vi "MAIN_cRIO_ZNB_AMI.vi"() -> ()   [LabVIEW 2017]
doc: "Use this template to build a producer/consumer design pattern with events to produce queue items. Use this design pattern instead of the user interface event handler pattern for user interfaces when you want to execute code asynchronously in response to an event without slowing the user interface responsiveness."
uses:
  MEDIDA_cRIO_ZNB_AMI_DATOS.ctl
  AMI MAGNET/Status AMI.ctl
  MAIN_cRIO_ZNB_AMI.ctl
  DISPLAY/UserEventData.ctl
  DISPLAY/DataType.ctl
  cRIO_ZNB_AMI_GLOBALES.vi
panel:
  out "X state":T1=1 items=["Unknown", "RAMPING to target field/current", "HOLDING at the target field/current", "PAUSED", "Ramping in MANUAL UP mode", "Ramping in MANUAL DOWN mode", "ZEROING CURRENT (in progress)", "Quench detected", "At ZERO current", "Heating persistent switch", "Cooling persistent switch", "External Rampdown active"]
  out "Y state":T1=1 items=["Unknown", "RAMPING to target field/current", "HOLDING at the target field/current", "PAUSED", "Ramping in MANUAL UP mode", "Ramping in MANUAL DOWN mode", "ZEROING CURRENT (in progress)", "Quench detected", "At ZERO current", "Heating persistent switch", "Cooling persistent switch", "External Rampdown active"]
  out "Z state":T1=1 items=["Unknown", "RAMPING to target field/current", "HOLDING at the target field/current", "PAUSED", "Ramping in MANUAL UP mode", "Ramping in MANUAL DOWN mode", "ZEROING CURRENT (in progress)", "Quench detected", "At ZERO current", "Heating persistent switch", "Cooling persistent switch", "External Rampdown active"]
  out "Temperature Status":i32(ring) items=["TemperatureUnknown", "Stable", "Tracking", "Near"]
  out "DataPath":path
  out "XY Graph 4":cluster{dbl[], dbl[]}[](graph)
  out "XY Graph 3":cluster{dbl[], dbl[]}[](graph)
  out "XY Graph 2":cluster{dbl[], dbl[]}[](graph)
  out "XY Graph 1":cluster{dbl[], dbl[]}[](graph)
  out "arrayDatos":T2[](array[typedef]) {"CampoZ(T)" format="%.3e"; "CampoY(T)" format="%.3e"; "A.Input3(V)" format="%.3e"; "A.Input4(V)" format="%.3e"; "A.Input1(V)" format="%.3e"; "A.Input2(V)" format="%.3e"; "Temperatura(K)" format="%.3e"; "CampoX(T)" format="%.3e"; "Tiempo(min)" format="%.3e"}
  out "Puntos":i32=10000
  out "Status":bool
  in  "Programa":i32(listbox)=-1
  in  "Setup":bool
  in  "Programar":bool
  in  "Fin":bool
  in  "Auto":bool
  in  "Parar":bool
  out "Tiempo(min)":dbl format="%.2f"
  out "A.Input2(V)":dbl format="%.3f"
  out "A.Input3(V)":dbl format="%.3f"
  out "A.Input4(V)":dbl format="%.3f"
  out "Campo Mag(T)":dbl format="%.2f"
  out "Temperatura(K)":dbl format="%.2f"
  out "TotalSeq":string[](array[string])
  in  "Grafica":T3(ring)
  out "Estado":string
  out "NumCommando":string
  in  "Pausa":bool
  in  "Saltar":bool
  out "Total Comandos":i32
  out "Comando actual":i32
  out "Datos":T2 {"CampoZ(T)" format="%.3e"; "CampoY(T)" format="%.3e"; "A.Input3(V)" format="%.3e"; "A.Input4(V)" format="%.3e"; "A.Input1(V)" format="%.3e"; "A.Input2(V)" format="%.3e"; "Temperatura(K)" format="%.3e"; "CampoX(T)" format="%.3e"; "Tiempo(min)" format="%.3e"}
  out "error out":errorcluster
  # "cRIO - 9074.ZNB.AMI\nEnero 2023 V1.0  a-sslcdms LV2017"
  # "Secuencia en marcha. Pulsar para PAUSAR"
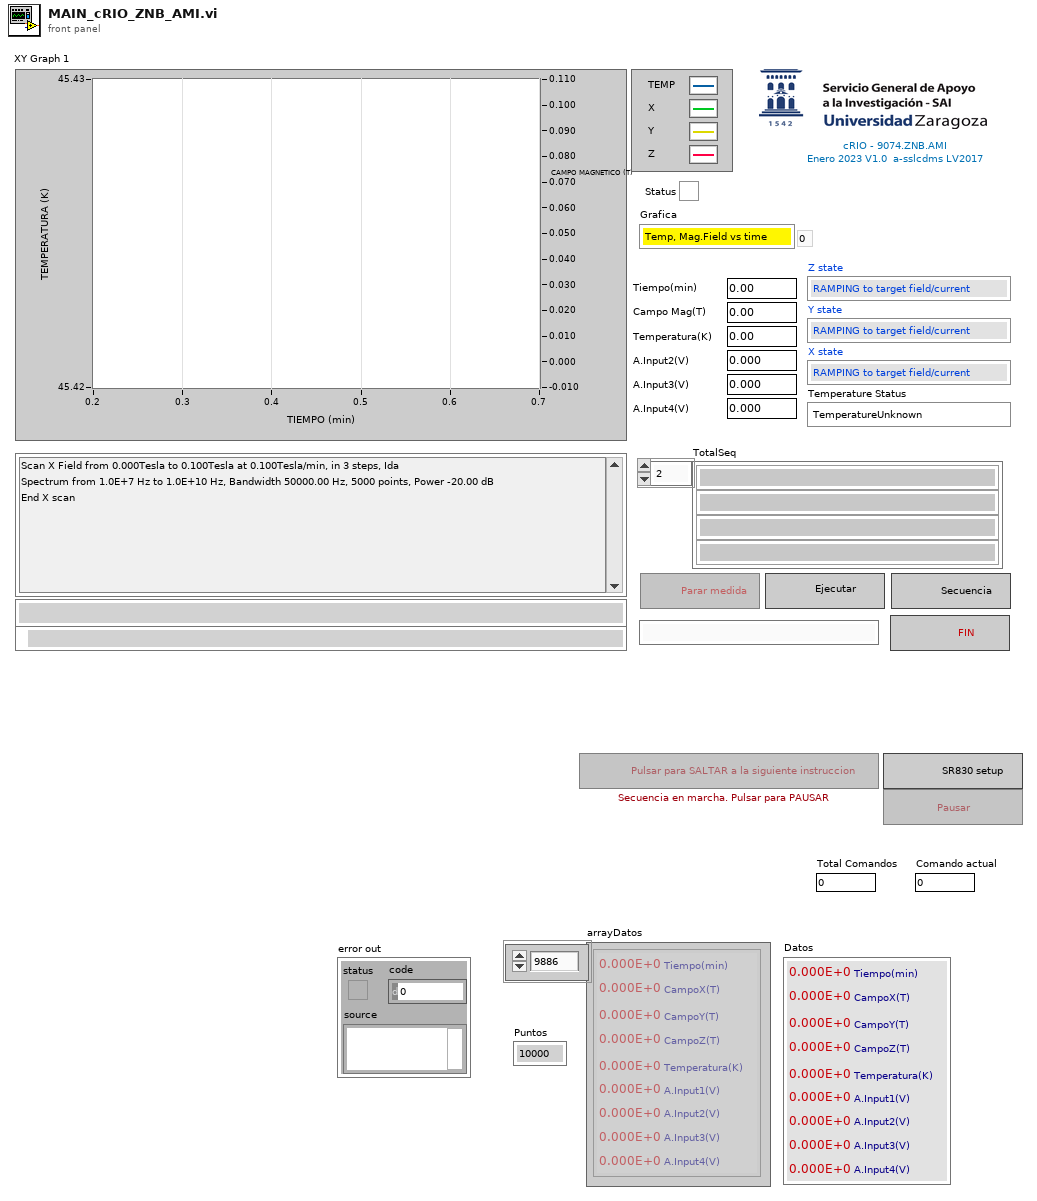
[diagram p1: front panel]
types:
  T1 = typedef "Status AMI.ctl" = u16
  T2 = typedef "MEDIDA_cRIO_ZNB_AMI_DATOS.ctl" = cluster{"Tiempo(min)":dbl, "CampoX(T)":dbl, "CampoY(T)":dbl, "CampoZ(T)":dbl, "Temperatura(K)":dbl, "A.Input1(V)":dbl, "A.Input2(V)":dbl, "A.Input3(V)":dbl, "A.Input4(V)":dbl}
  T3 = enum16{"Temp, Mag.Field vs time", "Voltajes 2,3,4 vs Tiempo", "Voltajes 2,3,4 vs Campo", "Voltajes 2,3,4 vs Temper."}
  T4 = typedef "UserEventData.ctl" = cluster{"DataType":T5, "Data":variant}
  T5 = typedef "DataType.ctl" = enum16{"Initialize Front Panel", "Update Front Panel", "Update Graph", "Enable/Disable Controls", "Update Status"}
  T6 = typedef "MAIN_cRIO_ZNB_AMI.ctl" = enum16{"Inicializar", "Ajustes", "Medir", "Finalizar"}
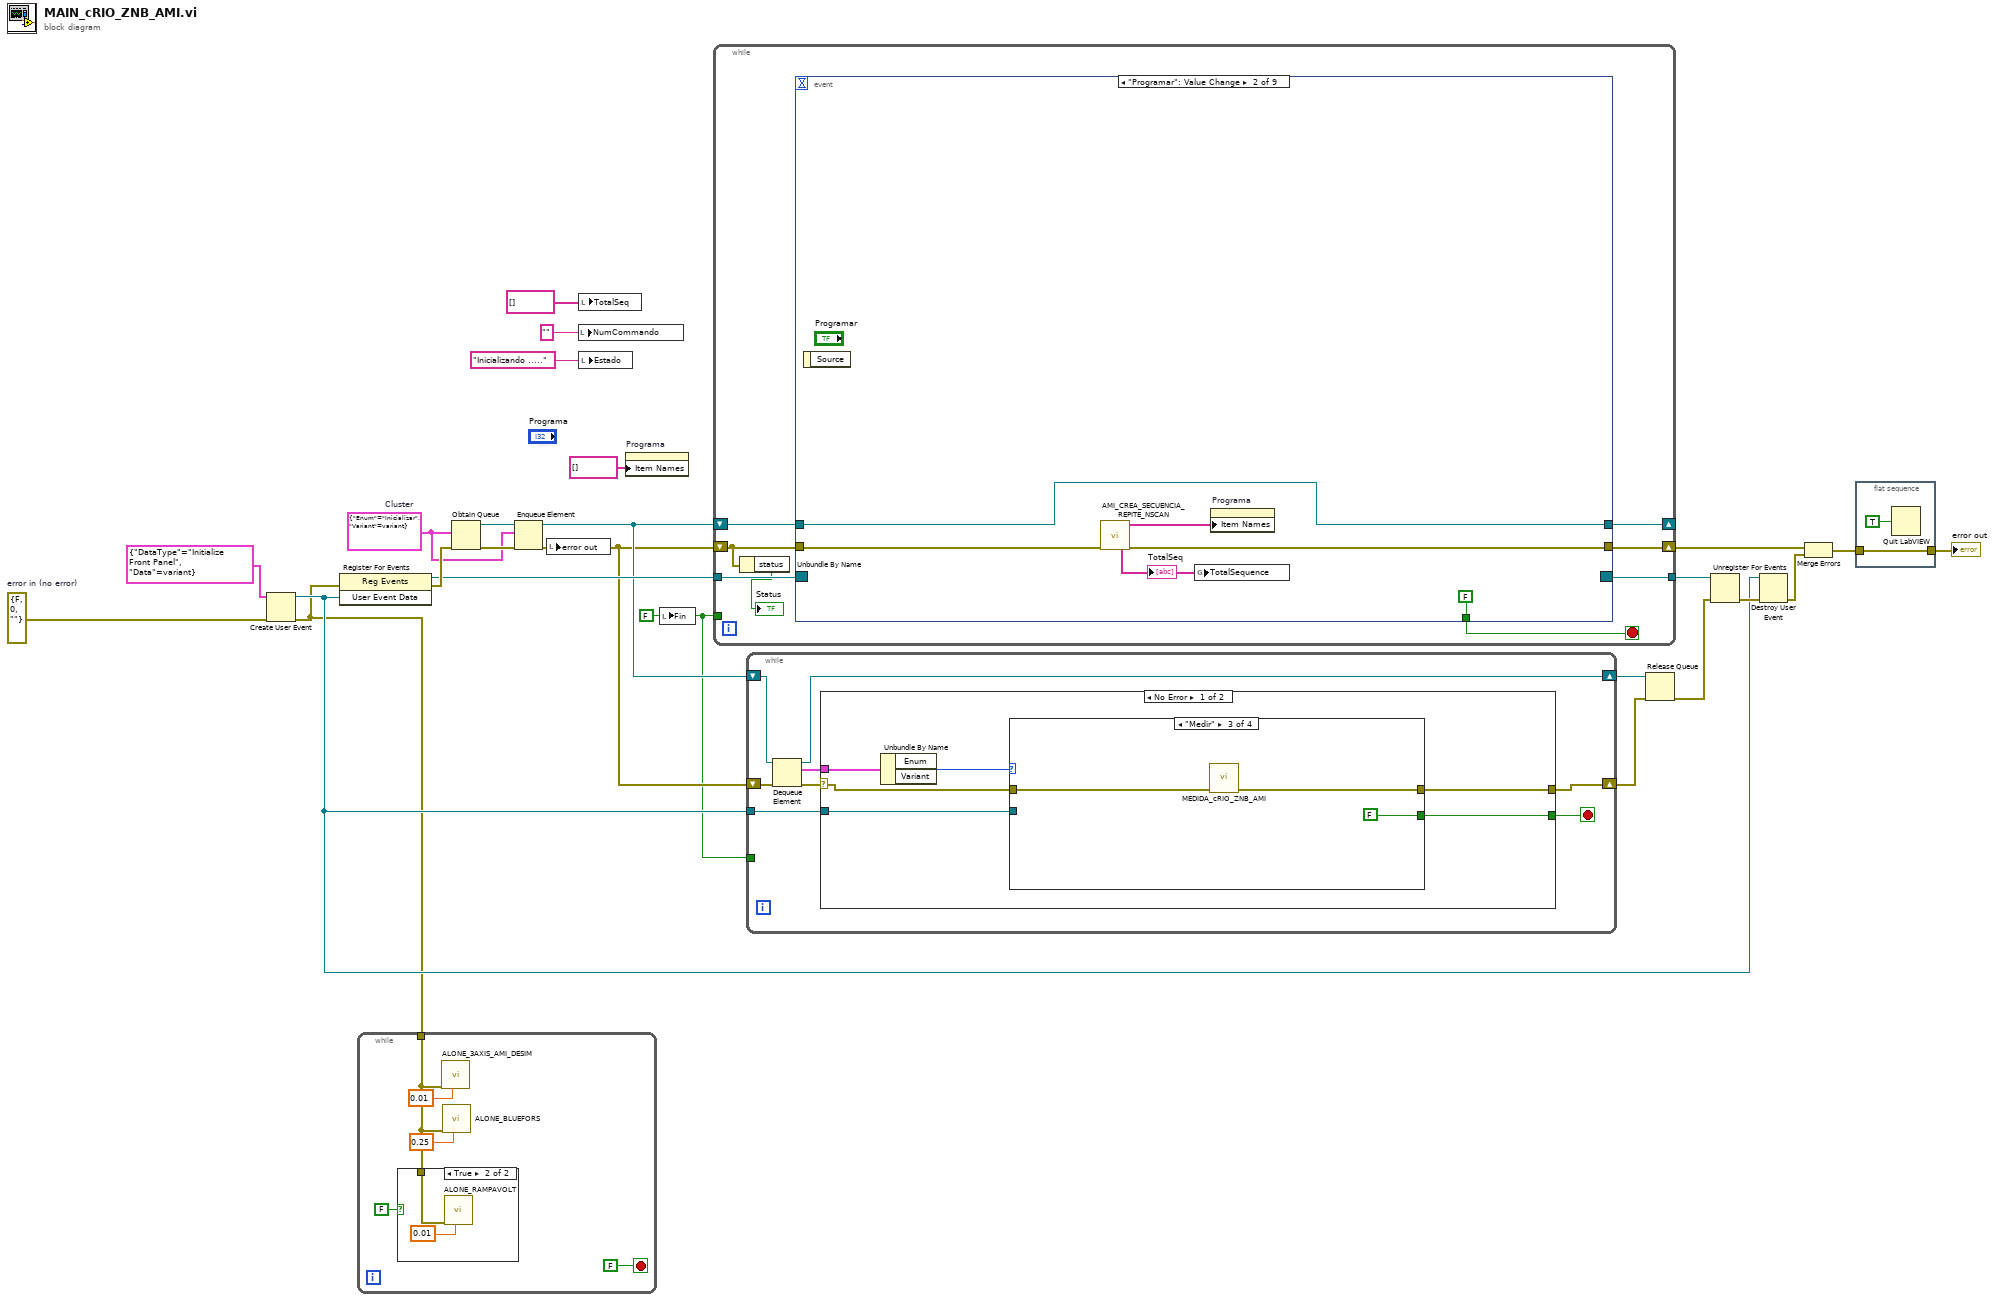
[diagram p0: block diagram]
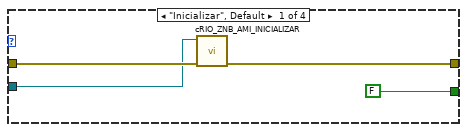
[diagram p3: hidden frame]
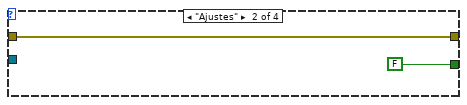
[diagram p4: hidden frame]
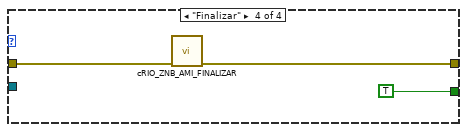
[diagram p5: hidden frame]
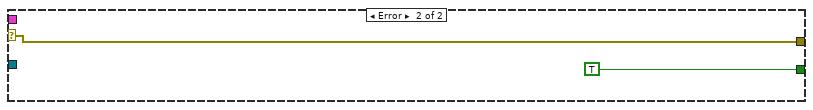
[diagram p6: hidden frame]
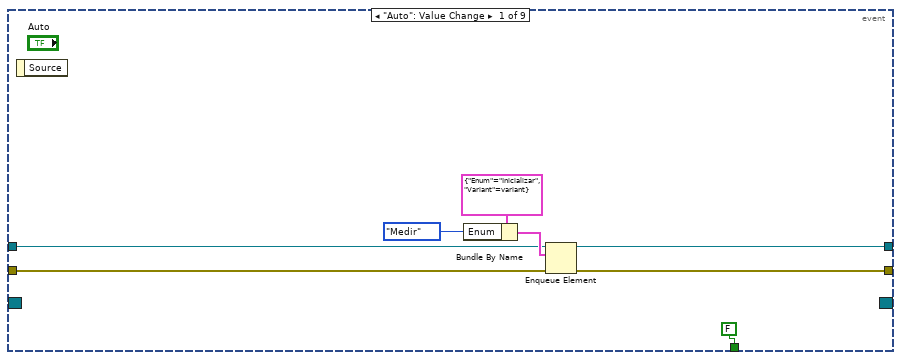
[diagram p7: hidden frame]
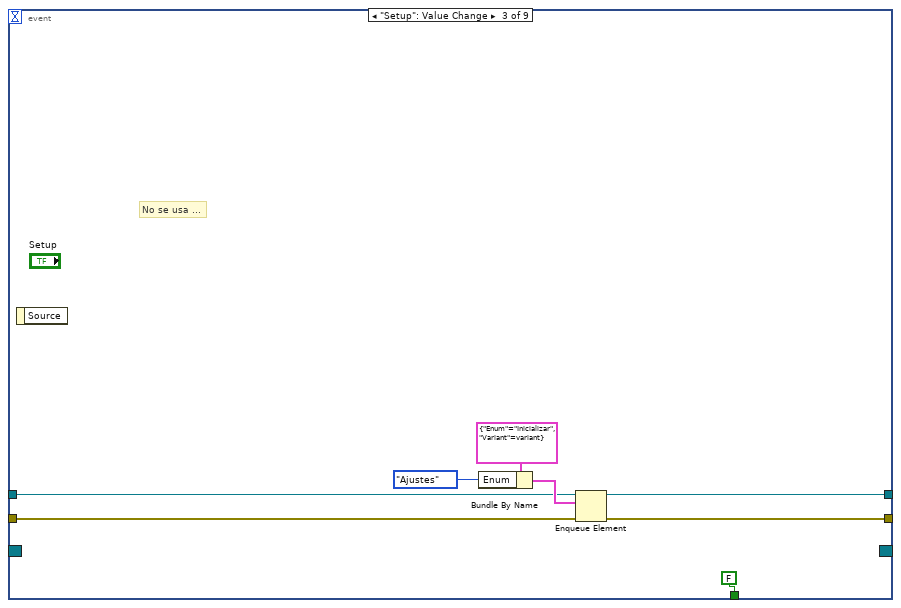
[diagram p8: hidden frame]
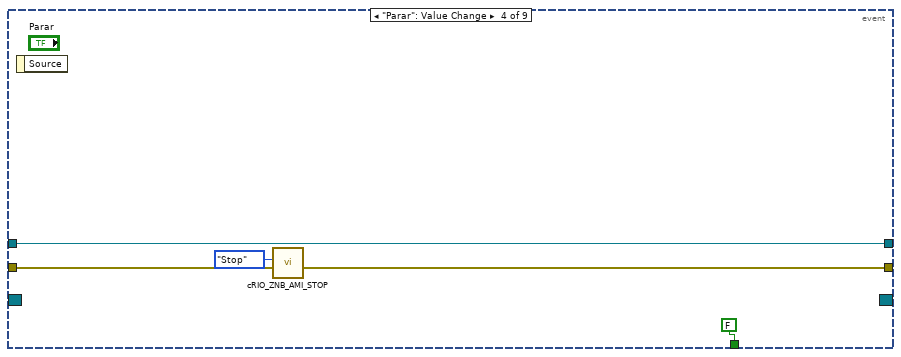
[diagram p9: hidden frame]
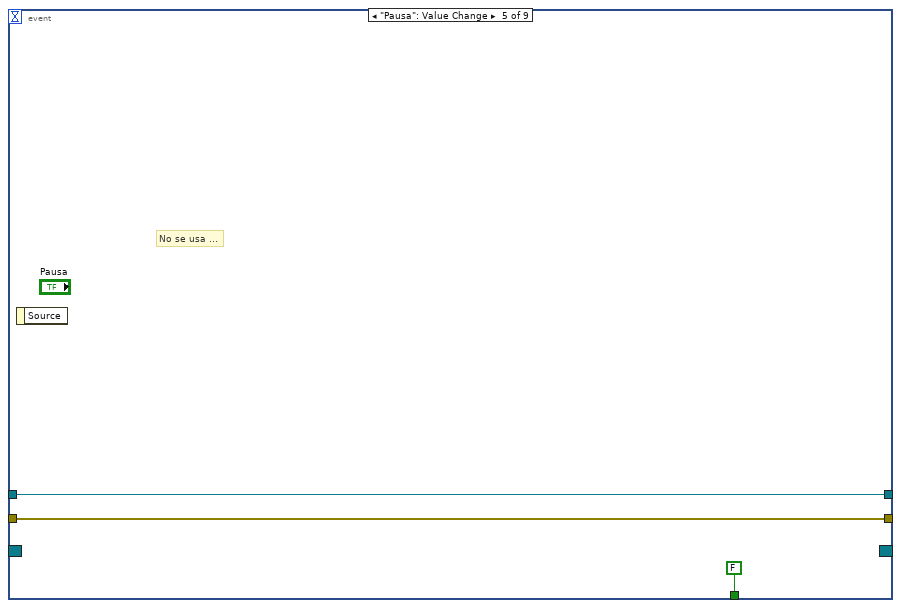
[diagram p10: hidden frame]
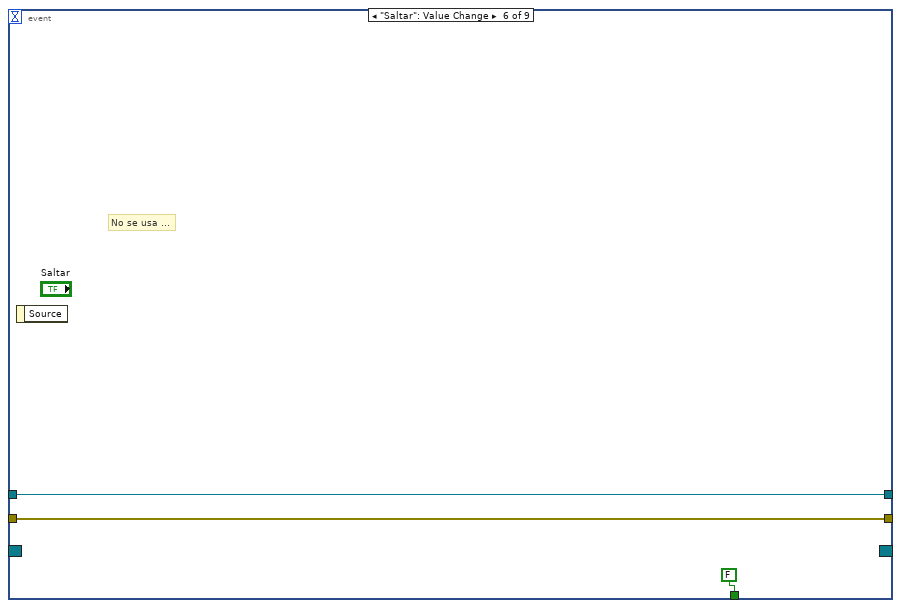
[diagram p11: hidden frame]
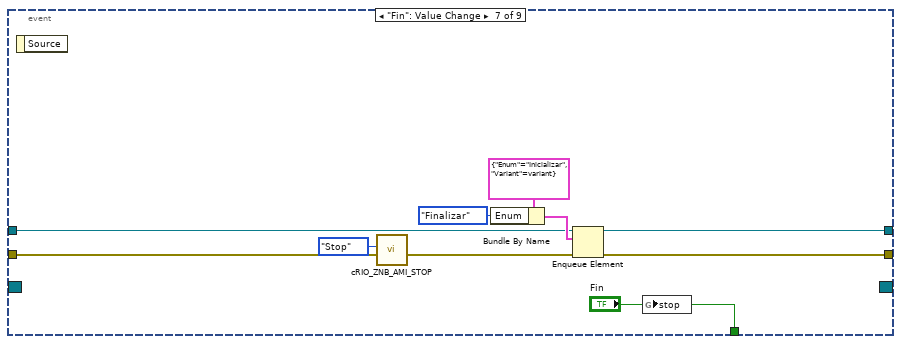
[diagram p12: hidden frame]
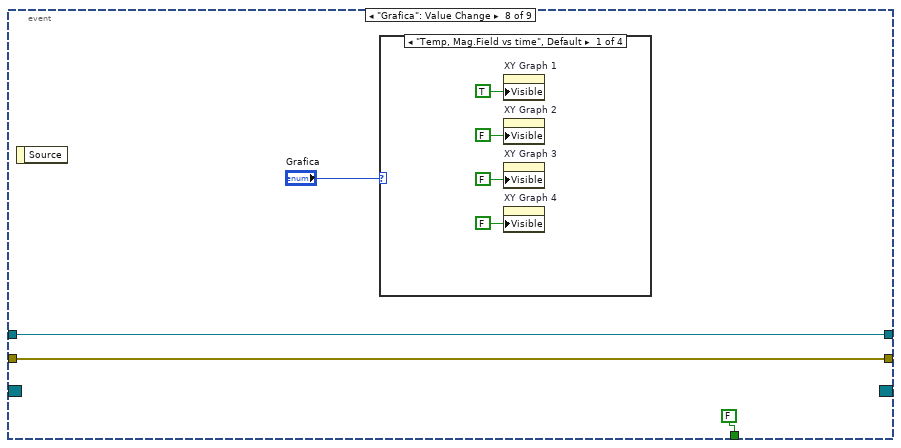
[diagram p13: hidden frame]
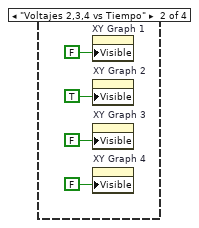
[diagram p14: hidden frame]
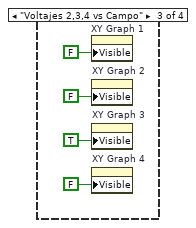
[diagram p15: hidden frame]
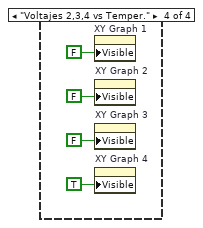
[diagram p16: hidden frame]
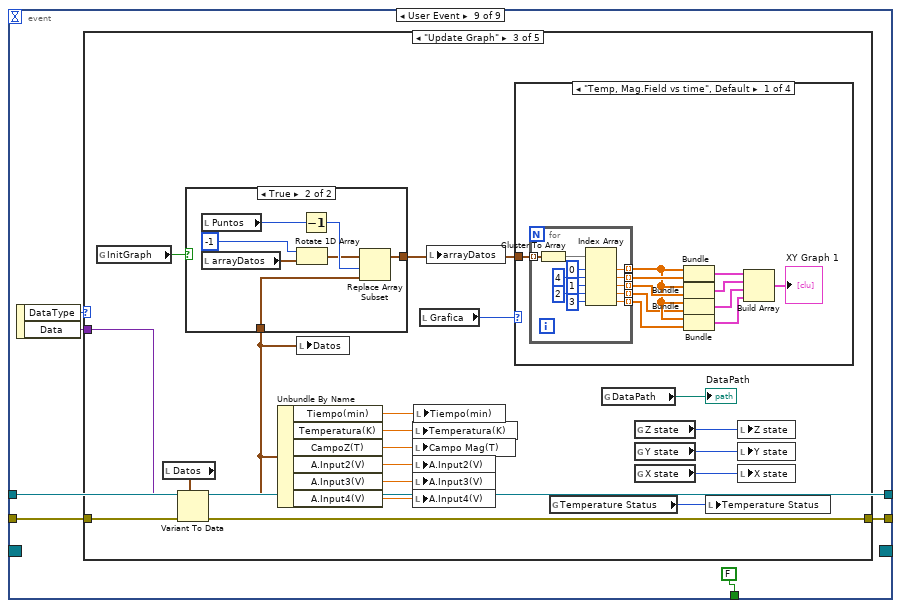
[diagram p17: hidden frame]
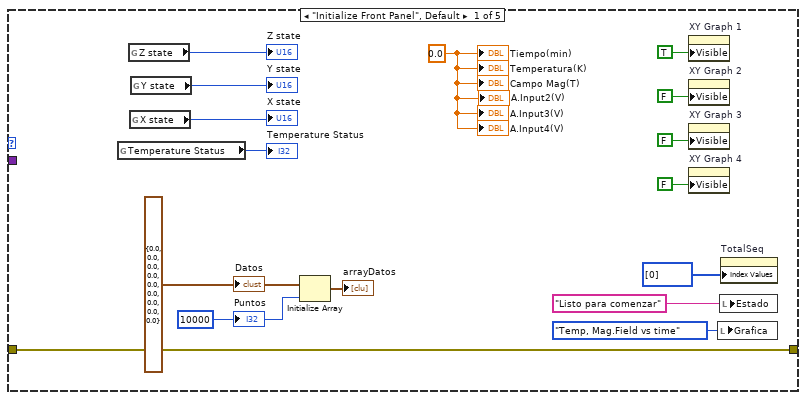
[diagram p18: hidden frame]
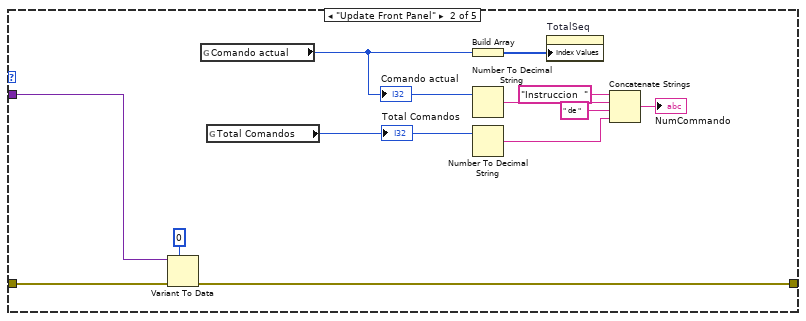
[diagram p19: hidden frame]
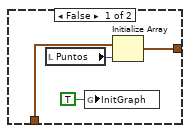
[diagram p20: hidden frame]
diagram:
  w5 = FALSE ("Fin")
  w2 = errorcluster {"status"=FALSE, "code"=0, "source"=""}  # error in (no error)
  w23 = cluster{"Enum":T6, "Variant":variant} {"Enum"=enum."Inicializar", "Variant"=variant}  # Cluster
  n1 = Create User Event(user event datatype=T4 {"DataType"=enum."Initialize Front Panel", "Data"=variant} ("User Event Data"), error in=w2) -> (user event=w11:refnum<user-event>, error out=w1:errorcluster)
  n2 = register-events(error in=w1, w11) -> (reference out=w15:refnum<event-registration>, error out=w25:errorcluster)  [unwired: 1 in]
  n3 = while {
    tunnel: w1 -> [w30]
    stop <- FALSE stop-if-true
    n4 = case shown="True" FALSE {
      tunnel: w30 -> [_ w32]
      frame False {
      }
      frame True {
        n5 = call "ALONE_RAMPAVOLT.vi"("Refresco(s)"=0.01, "error in (no error)"=w32) -> ()  [unwired: 8 in, 2 out]
      }
    }
    n6 = call "ALONE_3AXIS_AMI_DESIM.vi"("Refresco(s)"=0.01, "error in (no error)"=w30) -> ()  [unwired: 8 in, 2 out]
    n7 = call "ALONE_BLUEFORS.vi"("Refresco(s)"=0.25, "error in (no error)"=w30) -> ()  [unwired: 9 in, 1 out]
  }
  n8 = Obtain Queue(element data type=w23, error in (no error)=w25) -> (queue out=w22:refnum<queue>, error out=w24:errorcluster)  [unwired: 3 in, 1 out]
  n9 = Enqueue Element(queue=w22, element=w23, error in (no error)=w24) -> (queue out=w13:refnum<queue>, error out=w12:errorcluster)  [unwired: 1 in, 1 out]
  n10 = local write "error out"(w12) -> ()
  n11 = local write "NumCommando"("" ("NumCommando")) -> ()
  n12 = local write "TotalSeq"(string[] [] ("TotalSequence")) -> ()
  n13 = local write "Estado"("Inicializando ....." ("String")) -> ()
  n14 = property on="Programa" class="LstBox (strict)"("Item Names"=string[] []) -> ()  [unwired: 2 in, 2 out]
  n15 = local write "Fin"(w5) -> ()
  n16 = while {
    shift-right: [w35] -> w18
    shift-left: w12 -> [w34]
    shift-right: [w39] -> _
    shift-left: w13 -> [w40]
    tunnel: w15 -> [w37]
    tunnel: [w36] -> w14
    tunnel: w5 -> [_]
    stop <- w38 stop-if-true
    n17 = Unbundle By Name(w34) -> ("status"=→"Status":bool)
    n18 = event shown="[1] \"Programar\": Value Change" {
      selector: w37 -> [_ _ _ _ _ _ _ _ _]
      dyn-events: [_ _ _ _ _ _ _ _ _] -> w36
      timeout: _ -> [_ _ _ _ _ _ _ _ _]
      tunnel: w40 -> [w43 w51 w55 w64 w69 w72 w78 w85 w105]
      tunnel: [w44 w51 w57 w64 w69 w72 w79 w85 w105] -> w39
      tunnel: w34 -> [w42 w53 w56 w66 w68 w71 w76 w84 w107]
      tunnel: [w45 w52 w58 w63 w68 w71 w80 w84 w106] -> w35
      tunnel: [FALSE ("Parar") FALSE ("Parar") FALSE ("Parar") FALSE ("Parar") FALSE ("Parar") FALSE ("Parar") "Fin" FALSE ("Parar") FALSE ("Parar")] -> w38
      event "Auto": Value Change {
        n19 = event-data() -> ()  [unwired: 1 in, 1 out]
        n20 = Bundle By Name(cluster=cluster{"Enum":T6, "Variant":variant} {"Enum"=enum."Inicializar", "Variant"=variant} ("Cluster"), "Enum"=MAIN_cRIO_ZNB_AMI."Medir") -> (w46:cluster{"Enum":T6, "Variant":variant})
        n21 = Enqueue Element(queue=w43, element=w46, error in (no error)=w42) -> (queue out=w44:refnum<queue>, error out=w45:errorcluster)  [unwired: 1 in, 1 out]
      }
      event "Programar": Value Change {
        n22 = event-data() -> ()  [unwired: 1 in, 1 out]
        n23 = call "AMI_CREA_SECUENCIA_REPITE_NSCAN.vi"("error in (no error)"=w53) -> ("error out"=w52:errorcluster, "SECUENCIA"=w50:string[], "TOTAL_REPS"=w49:string[])  [unwired: 7 in, 1 out]
        "TotalSeq" <- w49
        n24 = global write "cRIO_ZNB_AMI_GLOBALES.vi" "TotalSequence"(w49) -> ()
        n25 = property on="Programa" class="LstBox (strict)"("Item Names"=w50) -> ()  [unwired: 2 in, 2 out]
      }
      event "Setup": Value Change {
        # "No se usa ..."
        n26 = event-data() -> ()  [unwired: 1 in, 1 out]
        n27 = Bundle By Name(cluster=cluster{"Enum":T6, "Variant":variant} {"Enum"=enum."Inicializar", "Variant"=variant} ("Cluster"), "Enum"=MAIN_cRIO_ZNB_AMI."Ajustes") -> (w59:cluster{"Enum":T6, "Variant":variant})
        n28 = Enqueue Element(queue=w55, element=w59, error in (no error)=w56) -> (queue out=w57:refnum<queue>, error out=w58:errorcluster)  [unwired: 1 in, 1 out]
      }
      event "Parar": Value Change {
        n29 = event-data() -> ()  [unwired: 1 in, 1 out]
        n30 = call "cRIO_ZNB_AMI_STOP.vi"("error in (no error)"=w66, "Stop"=enum16{"Continue", "Stop", "Default"}."Stop") -> ("error out"=w63:errorcluster)  [unwired: 8 in, 1 out]
      }
      event "Pausa": Value Change {
        # "No se usa ..."
        n31 = event-data() -> ()  [unwired: 1 in, 1 out]
      }
      event "Saltar": Value Change {
        # "No se usa ..."
        n32 = event-data() -> ()  [unwired: 1 in, 1 out]
      }
      event "Fin": Value Change {
        n33 = event-data() -> ()  [unwired: 1 in, 1 out]
        n34 = call "cRIO_ZNB_AMI_STOP.vi"("error in (no error)"=w76, "Stop"=enum16{"Continue", "Stop", "Default"}."Stop") -> ("error out"=w75:errorcluster)  [unwired: 8 in, 1 out]
        n35 = Bundle By Name(cluster=cluster{"Enum":T6, "Variant":variant} {"Enum"=enum."Inicializar", "Variant"=variant} ("Cluster"), "Enum"=MAIN_cRIO_ZNB_AMI."Finalizar") -> (w81:cluster{"Enum":T6, "Variant":variant})
        n36 = Enqueue Element(queue=w78, element=w81, error in (no error)=w75) -> (queue out=w79:refnum<queue>, error out=w80:errorcluster)  [unwired: 1 in, 1 out]
        n37 = global write "cRIO_ZNB_AMI_GLOBALES.vi" "stop"("Fin") -> ()
      }
      event "Grafica": Value Change {
        n38 = event-data() -> ()  [unwired: 1 in, 1 out]
        n39 = case shown="\"Temp, Mag.Field vs time\", Default" "Grafica" {
          frame "Temp, Mag.Field vs time", Default {
            n40 = property on="XY Graph 1" class="XYGraph (strict)"("Visible"=TRUE) -> ()  [unwired: 2 in, 2 out]
            n41 = property on="XY Graph 2" class="XYGraph (strict)"("Visible"=FALSE) -> ()  [unwired: 2 in, 2 out]
            n42 = property on="XY Graph 3" class="XYGraph (strict)"("Visible"=FALSE) -> ()  [unwired: 2 in, 2 out]
            n43 = property on="XY Graph 4" class="XYGraph (strict)"("Visible"=FALSE) -> ()  [unwired: 2 in, 2 out]
          }
          frame "Voltajes 2,3,4 vs Tiempo" {
            n44 = property on="XY Graph 1" class="XYGraph (strict)"("Visible"=FALSE) -> ()  [unwired: 2 in, 2 out]
            n45 = property on="XY Graph 2" class="XYGraph (strict)"("Visible"=TRUE) -> ()  [unwired: 2 in, 2 out]
            n46 = property on="XY Graph 3" class="XYGraph (strict)"("Visible"=FALSE) -> ()  [unwired: 2 in, 2 out]
            n47 = property on="XY Graph 4" class="XYGraph (strict)"("Visible"=FALSE) -> ()  [unwired: 2 in, 2 out]
          }
          frame "Voltajes 2,3,4 vs Campo" {
            n48 = property on="XY Graph 1" class="XYGraph (strict)"("Visible"=FALSE) -> ()  [unwired: 2 in, 2 out]
            n49 = property on="XY Graph 2" class="XYGraph (strict)"("Visible"=FALSE) -> ()  [unwired: 2 in, 2 out]
            n50 = property on="XY Graph 3" class="XYGraph (strict)"("Visible"=TRUE) -> ()  [unwired: 2 in, 2 out]
            n51 = property on="XY Graph 4" class="XYGraph (strict)"("Visible"=FALSE) -> ()  [unwired: 2 in, 2 out]
          }
          frame "Voltajes 2,3,4 vs Temper." {
            n52 = property on="XY Graph 1" class="XYGraph (strict)"("Visible"=FALSE) -> ()  [unwired: 2 in, 2 out]
            n53 = property on="XY Graph 2" class="XYGraph (strict)"("Visible"=FALSE) -> ()  [unwired: 2 in, 2 out]
            n54 = property on="XY Graph 3" class="XYGraph (strict)"("Visible"=FALSE) -> ()  [unwired: 2 in, 2 out]
            n55 = property on="XY Graph 4" class="XYGraph (strict)"("Visible"=TRUE) -> ()  [unwired: 2 in, 2 out]
          }
        }
      }
      event User Event {
        n56 = event-data() -> ("DataType"=w109:T5, "Data"=w108:variant)  [unwired: 1 in]
        n57 = case shown="\"Update Graph\"" w109 {
          tunnel: w108 -> [_ w135 w155 w251 w274]
          tunnel: w107 -> [w125 w136 w156 w254 w273]
          tunnel: [w125 w129 w153 w253 w272] -> w106
          frame "Initialize Front Panel", Default {
            w113 = 0.0 ("Tiempo(min)")
            w116 = T2 {"Tiempo(min)"=0.0, "CampoX(T)"=0.0, "CampoY(T)"=0.0, "CampoZ(T)"=0.0, "Temperatura(K)"=0.0, "A.Input1(V)"=0.0, "A.Input2(V)"=0.0, "A.Input3(V)"=0.0, "A.Input4(V)"=0.0} ("Datos")
            w117 = 10000 ("Puntos")
            n58 = global read "cRIO_ZNB_AMI_GLOBALES.vi" "Temperature Status"() -> (→"Temperature Status":i32)
            n59 = global read "cRIO_ZNB_AMI_GLOBALES.vi" "Z state"() -> (→"Z state":T1)
            n60 = global read "cRIO_ZNB_AMI_GLOBALES.vi" "X state"() -> (→"X state":T1)
            n61 = global read "cRIO_ZNB_AMI_GLOBALES.vi" "Y state"() -> (→"Y state":T1)
            n62 = Initialize Array(w116, w117) -> (→"arrayDatos":T2[])
            n63 = property on="XY Graph 1" class="XYGraph (strict)"("Visible"=TRUE) -> ()  [unwired: 2 in, 2 out]
            n64 = property on="XY Graph 2" class="XYGraph (strict)"("Visible"=FALSE) -> ()  [unwired: 2 in, 2 out]
            n65 = property on="XY Graph 3" class="XYGraph (strict)"("Visible"=FALSE) -> ()  [unwired: 2 in, 2 out]
            n66 = property on="XY Graph 4" class="XYGraph (strict)"("Visible"=FALSE) -> ()  [unwired: 2 in, 2 out]
            n67 = local write "Grafica"(T3."Temp, Mag.Field vs time" ("Grafica")) -> ()
            n68 = local write "Estado"("Listo para comenzar" ("String")) -> ()
            n69 = property on="TotalSeq" class="Arr (strict)"("Index Values"=u32[] [0]) -> ()  [unwired: 2 in, 2 out]
            "Puntos" <- w117
            "Tiempo(min)" <- w113
            "A.Input3(V)" <- w113
            "A.Input4(V)" <- w113
            "Campo Mag(T)" <- w113
            "Temperatura(K)" <- w113
            "Datos" <- w116
            "A.Input2(V)" <- w113
          }
          frame "Update Front Panel" {
            n70 = Variant To Data(error in=w136, type=0, Variant=w135) -> (error out=w129:errorcluster)  [unwired: 1 out]
            n71 = global read "cRIO_ZNB_AMI_GLOBALES.vi" "Comando actual"() -> (w126:i32)
            "Comando actual" <- w126
            n72 = global read "cRIO_ZNB_AMI_GLOBALES.vi" "Total Comandos"() -> (w127:i32)
            "Total Comandos" <- w127
            n73 = Build Array(w126) -> (w128:i32[])
            n74 = Number To Decimal String(number=w126) -> (decimal integer string=w133:string)  [unwired: 1 in]
            n75 = Number To Decimal String(number=w127) -> (decimal integer string=w131:string)  [unwired: 1 in]
            n76 = property on="TotalSeq" class="Arr (strict)"("Index Values"=w128) -> ()  [unwired: 2 in, 2 out]
            n77 = Concatenate Strings("Instruccion  " ("string"), w133, " de " ("string"), w131) -> (→"NumCommando":string)
          }
          frame "Update Graph" {
            n78 = global read "cRIO_ZNB_AMI_GLOBALES.vi" "InitGraph"() -> (w141:bool)
            n79 = local read "Datos"() -> (w154:T2)
            n80 = Variant To Data(error in=w156, type=w154, Variant=w155) -> (data=w143:T2, error out=w153:errorcluster)
            n81 = case shown="True" w141 {
              tunnel: [w157 w162] -> w151
              tunnel: w143 -> [w158 w161]
              frame False {
                n82 = local read "Puntos"() -> (w159:i32)
                n83 = global write "cRIO_ZNB_AMI_GLOBALES.vi" "InitGraph"(TRUE ("InitGraph")) -> ()
                n84 = Initialize Array(w158, w159) -> (w157:T2[])
              }
              frame True {
                n85 = local read "Puntos"() -> (w166:i32)
                n86 = local read "arrayDatos"() -> (w163:T2[])
                n87 = Rotate 1D Array(1:w163, 2:-1 ("n")) -> (0:w165:T2[])
                n88 = Decrement(x=w166) -> (x-1=w167:i32)
                n89 = Replace Array Subset(array=w165, new element=w161, index=w167) -> (w162:T2[])
              }
            }
            n90 = Unbundle By Name(w143) -> ("Tiempo(min)"=w149:dbl, "Temperatura(K)"=w144:dbl, "CampoZ(T)"=w145:dbl, "A.Input2(V)"=w147:dbl, "A.Input3(V)"=w148:dbl, "A.Input4(V)"=w146:dbl)
            n91 = local write "Datos"(w143) -> ()
            n92 = local write "Temperatura(K)"(w144) -> ()
            n93 = local write "Campo Mag(T)"(w145) -> ()
            n94 = local write "A.Input2(V)"(w147) -> ()
            n95 = local write "A.Input3(V)"(w148) -> ()
            n96 = local write "A.Input4(V)"(w146) -> ()
            n97 = local write "Tiempo(min)"(w149) -> ()
            n98 = local read "Grafica"() -> (w152:T3)
            n99 = local write "arrayDatos"(w151) -> ()
            n100 = case shown="\"Temp, Mag.Field vs time\", Default" w152 {
              tunnel: w151 -> [w178 w199 w211 w230]
              frame "Temp, Mag.Field vs time", Default {
                n101 = for {
                  tunnel: w178 -> [w187] mode=indexing
                  tunnel: [w185] -> w172 mode=indexing
                  tunnel: [w184] -> w174 mode=indexing
                  tunnel: [w183] -> w173 mode=indexing
                  tunnel: [w182] -> w168 mode=indexing
                  tunnel: [w181] -> w169 mode=indexing
                  n102 = Cluster To Array(cluster=w187) -> (array=w186:dbl[])
                  n103 = Index Array(array=w186, index #1=0 ("index (row)"), index #2=4 ("index (row)"), index #3=1 ("index (row)"), index #4=2 ("index (row)"), index #5=3 ("index (row)")) -> (element #1=w185:dbl, element #2=w184:dbl, element #3=w183:dbl, element #4=w182:dbl, element #5=w181:dbl)
                }
                n104 = Bundle(w172, w174) -> (w177:cluster{dbl[], dbl[]})  [unwired: 1 in]
                n105 = Bundle(w172, w173) -> (w176:cluster{dbl[], dbl[]})  [unwired: 1 in]
                n106 = Bundle(w172, w168) -> (w171:cluster{dbl[], dbl[]})  [unwired: 1 in]
                n107 = Bundle(w172, w169) -> (w170:cluster{dbl[], dbl[]})  [unwired: 1 in]
                n108 = Build Array(w177, w176, w171, w170) -> (→"XY Graph 1":cluster{dbl[], dbl[]}[])
              }
              frame "Voltajes 2,3,4 vs Tiempo" {
                n109 = for {
                  tunnel: w199 -> [w206] mode=indexing
                  tunnel: [w204] -> w192 mode=indexing
                  tunnel: [w203] -> w196 mode=indexing
                  tunnel: [w202] -> w195 mode=indexing
                  tunnel: [w200] -> w193 mode=indexing
                  n110 = Cluster To Array(cluster=w206) -> (array=w205:dbl[])
                  n111 = Index Array(array=w205, index #1=0 ("index (row)"), index #2=6 ("index (row)"), index #3=7 ("index (row)"), index #4=8 ("index (row)")) -> (element #1=w204:dbl, element #2=w203:dbl, element #3=w202:dbl, element #4=w200:dbl)
                }
                n112 = Bundle(w192, w196) -> (w198:cluster{dbl[], dbl[]})  [unwired: 1 in]
                n113 = Bundle(w192, w195) -> (w197:cluster{dbl[], dbl[]})  [unwired: 1 in]
                n114 = Bundle(w192, w193) -> (w191:cluster{dbl[], dbl[]})  [unwired: 1 in]
                n115 = Build Array(w198, w197, w191) -> (→"XY Graph 2":cluster{dbl[], dbl[]}[])
              }
              frame "Voltajes 2,3,4 vs Campo" {
                n116 = for {
                  tunnel: w211 -> [w225] mode=indexing
                  tunnel: [w223] -> w213 mode=indexing
                  tunnel: [w222] -> w216 mode=indexing
                  tunnel: [w221] -> w215 mode=indexing
                  tunnel: [w219] -> w214 mode=indexing
                  n117 = Cluster To Array(cluster=w225) -> (array=w224:dbl[])
                  n118 = Index Array(array=w224, index #1=3 ("index (row)"), index #2=6 ("index (row)"), index #3=7 ("index (row)"), index #4=8 ("index (row)")) -> (element #1=w223:dbl, element #2=w222:dbl, element #3=w221:dbl, element #4=w219:dbl)
                }
                n119 = Bundle(w213, w216) -> (w218:cluster{dbl[], dbl[]})  [unwired: 1 in]
                n120 = Bundle(w213, w215) -> (w217:cluster{dbl[], dbl[]})  [unwired: 1 in]
                n121 = Bundle(w213, w214) -> (w212:cluster{dbl[], dbl[]})  [unwired: 1 in]
                n122 = Build Array(w218, w217, w212) -> (→"XY Graph 3":cluster{dbl[], dbl[]}[])
              }
              frame "Voltajes 2,3,4 vs Temper." {
                n123 = for {
                  tunnel: w230 -> [w244] mode=indexing
                  tunnel: [w242] -> w232 mode=indexing
                  tunnel: [w241] -> w235 mode=indexing
                  tunnel: [w240] -> w234 mode=indexing
                  tunnel: [w238] -> w233 mode=indexing
                  n124 = Cluster To Array(cluster=w244) -> (array=w243:dbl[])
                  n125 = Index Array(array=w243, index #1=4 ("index (row)"), index #2=6 ("index (row)"), index #3=7 ("index (row)"), index #4=8 ("index (row)")) -> (element #1=w242:dbl, element #2=w241:dbl, element #3=w240:dbl, element #4=w238:dbl)
                }
                n126 = Bundle(w232, w235) -> (w237:cluster{dbl[], dbl[]})  [unwired: 1 in]
                n127 = Bundle(w232, w234) -> (w236:cluster{dbl[], dbl[]})  [unwired: 1 in]
                n128 = Bundle(w232, w233) -> (w231:cluster{dbl[], dbl[]})  [unwired: 1 in]
                n129 = Build Array(w237, w236, w231) -> (→"XY Graph 4":cluster{dbl[], dbl[]}[])
              }
            }
            n130 = global read "cRIO_ZNB_AMI_GLOBALES.vi" "Temperature Status"() -> (w150:i32)
            n131 = global read "cRIO_ZNB_AMI_GLOBALES.vi" "DataPath"() -> (→"DataPath":path)
            n132 = global read "cRIO_ZNB_AMI_GLOBALES.vi" "Z state"() -> (w138:T1)
            n133 = global read "cRIO_ZNB_AMI_GLOBALES.vi" "Y state"() -> (w139:T1)
            n134 = global read "cRIO_ZNB_AMI_GLOBALES.vi" "X state"() -> (w140:T1)
            n135 = local write "Temperature Status"(w150) -> ()
            n136 = local write "Z state"(w138) -> ()
            n137 = local write "Y state"(w139) -> ()
            n138 = local write "X state"(w140) -> ()
          }
          frame "Enable/Disable Controls" {
            n139 = Variant To Data(error in=w254, type=0, Variant=w251) -> (data=w250:i32, error out=w253:errorcluster)
            n140 = property on="Saltar" class="Bool"("Disabled"=u8 2) -> ()  [unwired: 2 in, 2 out]
            n141 = property on="Pausa" class="Bool (strict)"("Disabled"=u8 2) -> ()  [unwired: 2 in, 2 out]
            n142 = case shown="2" w250 {
              frame 0, Default {
                # "Programa en pausa"
                n143 = property on="Setup" class="Bool"("Disabled"=u8 0) -> ()  [unwired: 2 in, 2 out]
                n144 = property on="Programar" class="Bool"("Disabled"=u8 0) -> ()  [unwired: 2 in, 2 out]
                n145 = property on="Auto" class="Bool"("Disabled"=u8 0) -> ()  [unwired: 2 in, 2 out]
                n146 = property on="Parar" class="Bool"("Disabled"=u8 2) -> ()  [unwired: 2 in, 2 out]
                n147 = property on="Fin" class="Bool (strict)"("Disabled"=u8 0) -> ()  [unwired: 2 in, 2 out]
              }
              frame 1 {
                # "Programa en manual"
                n148 = property on="Setup" class="Bool"("Disabled"=u8 0) -> ()  [unwired: 2 in, 2 out]
                n149 = property on="Programar" class="Bool"("Disabled"=u8 2) -> ()  [unwired: 2 in, 2 out]
                n150 = property on="Auto" class="Bool"("Disabled"=u8 2) -> ()  [unwired: 2 in, 2 out]
                n151 = property on="Parar" class="Bool"("Disabled"=u8 0) -> ()  [unwired: 2 in, 2 out]
                n152 = property on="Fin" class="Bool (strict)"("Disabled"=u8 2) -> ()  [unwired: 2 in, 2 out]
              }
              frame 2 {
                # "Programa en automatico"
                n153 = property on="Setup" class="Bool"("Disabled"=u8 0) -> ()  [unwired: 2 in, 2 out]
                n154 = property on="Programar" class="Bool"("Disabled"=u8 2) -> ()  [unwired: 2 in, 2 out]
                n155 = property on="Auto" class="Bool"("Disabled"=u8 2) -> ()  [unwired: 2 in, 2 out]
                n156 = property on="Parar" class="Bool"("Disabled"=u8 0) -> ()  [unwired: 2 in, 2 out]
                n157 = property on="Fin" class="Bool (strict)"("Disabled"=u8 2) -> ()  [unwired: 2 in, 2 out]
              }
            }
          }
          frame "Update Status" {
            n158 = Variant To Data(error in=w273, type=" ", Variant=w274) -> (data=→"Estado":string, error out=w272:errorcluster)
          }
        }
      }
    }
  }
  n159 = while {
    shift-right: [w280] -> w17
    shift-left: w13 -> [w282]
    shift-right: [w276] -> w16
    shift-left: w12 -> [w281]
    tunnel: w11 -> [w275]
    tunnel: w5 -> [_]
    stop <- w278 stop-if-true
    n160 = Dequeue Element(queue=w282, error in (no error)=w281) -> (queue out=w280:refnum<queue>, element=w277:cluster{"Enum":T6, "Variant":variant}, error out=w279:errorcluster)  [unwired: 1 in, 1 out]
    n161 = case shown="No Error" w279 {
      selector: w279 -> [w286 w301]
      tunnel: [w284 TRUE] -> w278
      tunnel: w277 -> [w288 _]
      tunnel: [w285 w301] -> w276
      tunnel: w275 -> [w283 _]
      frame No Error {
        n162 = Unbundle By Name(w288) -> ("Enum"=w287:T6)  [unwired: 1 out]
        n163 = case shown="\"Medir\"" w287 {
          tunnel: w286 -> [w290 w293 w296 w299]
          tunnel: [w291 w293 w295 w298] -> w285
          tunnel: [FALSE FALSE FALSE TRUE] -> w284
          tunnel: w283 -> [w289 _ _ _]
          frame "Inicializar", Default {
            n164 = call "cRIO_ZNB_AMI_INICIALIZAR.vi"("error in (no error)"=w290, "User event"=w289) -> ("error out"=w291:errorcluster)  [unwired: 9 in]
          }
          frame "Ajustes" {
          }
          frame "Medir" {
            n165 = call "MEDIDA_cRIO_ZNB_AMI.vi"("error in (no error)"=w296) -> ("error out"=w295:errorcluster)  [unwired: 10 in]
          }
          frame "Finalizar" {
            n166 = call "cRIO_ZNB_AMI_FINALIZAR.vi"("error in (no error)"=w299) -> ("error out"=w298:errorcluster)  [unwired: 10 in]
          }
        }
      }
      frame Error {
      }
    }
  }
  n167 = Release Queue(queue=w17, error in (no error)=w16) -> (error out=w19:errorcluster)  [unwired: 1 in, 2 out]
  n168 = Unregister For Events(event registration refnum=w14, error in=w19) -> (error out=w20:errorcluster)
  n169 = Destroy User Event(user event=w11, error in=w20) -> (error out=w21:errorcluster)
  n170 = Merge Errors(w18, w21) -> (w10:errorcluster)
  n171 = flat-sequence {
    tunnel: w10 -> [w304]
    tunnel: [w304] -> w9
    frame #0 {
      n172 = Quit LabVIEW(quit? (T)=TRUE) -> ()
    }
  }
  "error out" <- w9
